vi "frontp_DO_replace_subpanel.vi"(8 "error in (no error)":errorcluster, 10 "changed_subpanel":refnum<vi>, 11 "front_panel in":refnum<class "front_panel.lvclass">) -> (0 "error out":errorcluster, 3 "front_panel out":refnum<class "front_panel.lvclass">)   [LabVIEW 2015, in "front_panel.lvclass"]
uses:
  front_panel.lvclass
  Hardware Class/hardware/hardware.lvclass
  hardware_caller_queue_numbers.ctl
  <vilib>/ActorFramework/Message Enqueuer/Message Enqueuer.lvclass/Message Enqueuer.ctl
  panel_class/panel.lvclass/panel.ctl
  stage_types.ctl
  Hardware Class/hardware_panel/Hardware_panel.lvclass
  Stage Class/Newport XPS/xps_panel/newport_xps_panel.lvclass
  Stage Class/Galvos_usb6212/galvo_panel/galvo_panel.lvclass
  Stage Class/Thorlabs Kinesis/thorlabs_panel/thorlabs_panel.lvclass
  Stage Class/MCL_3d200/mcl_panel.lvclass
  experiment_types.ctl
  Experiment/experiment_panel/Scan/scan_panel.lvclass
  Experiment/experiment_panel/2d_scan/scan_2d.lvclass
  Experiment/experiment_panel/PCFS/pcfs.lvclass
  detector_types.ctl
  Detector_Class/Picoquant/Hydraharp/hydraharp_panel/hydraharp_panel.lvclass
  Detector_Class/Picoquant/Picoharp/picoharp_panel/picoharp_panel.lvclass
  Detector_Class/Lightfield/lightfield_panel/lightfield_panel.lvclass
  <vilib>/ActorFramework/Message Enqueuer/Enqueue.vi
  <vilib>/ActorFramework/Message Priority Queue/Priority Enqueue.vi
  <vilib>/ActorFramework/Stop Msg/Stop Msg.lvclass
  panel_class/panel.lvclass
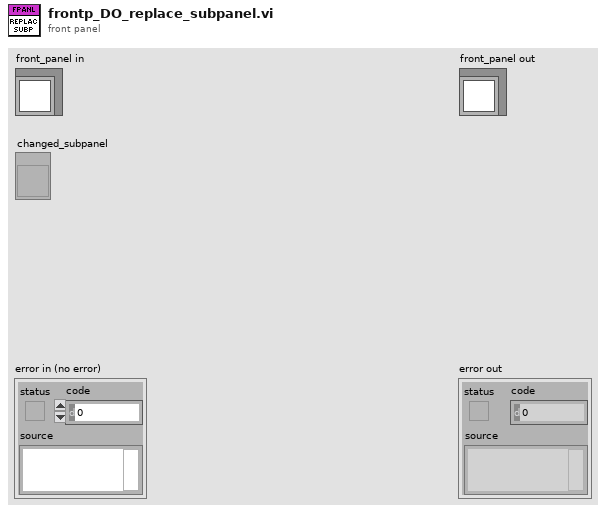
[diagram p1: front panel]
types:
  T1 = typedef "hardware_caller_queue_numbers.ctl" = enum16{"stage1", "stage2", "experiment", "detector"}
  T2 = typedef "stage_types.ctl" = enum16{"default", "Newport XPS", "Aerotech Ensemble", "Galvos", "Throlabs Kinesis", "MCL XYZ Piezo"}
  T3 = typedef "experiment_types.ctl" = enum16{"default", "PCFS", "Scan", "2D Galvo Scan"}
  T4 = typedef "detector_types.ctl" = enum16{"default", "Hydraharp", "Picoharp", "Lightfield"}
  T5 = typedef "ui_elements.ctl" = cluster{"map_xcursor":refnum<vi>, "map_ycursor":refnum<vi>}
  T6 = typedef "hardware_seqs.ctl" = refnum<queue>[]
  T7 = typedef "ui_plot_references.ctl" = cluster{"plots":refnum<vi>, "chart":refnum<vi>, "graph":refnum<vi>, "map":refnum<vi>, "XY Graph":refnum<vi>}
  T8 = typedef "ui_user_events.ctl" = cluster{"update_xy_graph":refnum<user-event>, "update_graph":refnum<user-event>, "update_chart":refnum<user-event>, "update_map":refnum<user-event>, "event_loop_stop":refnum<user-event>, "keep_map":refnum<user-event>}
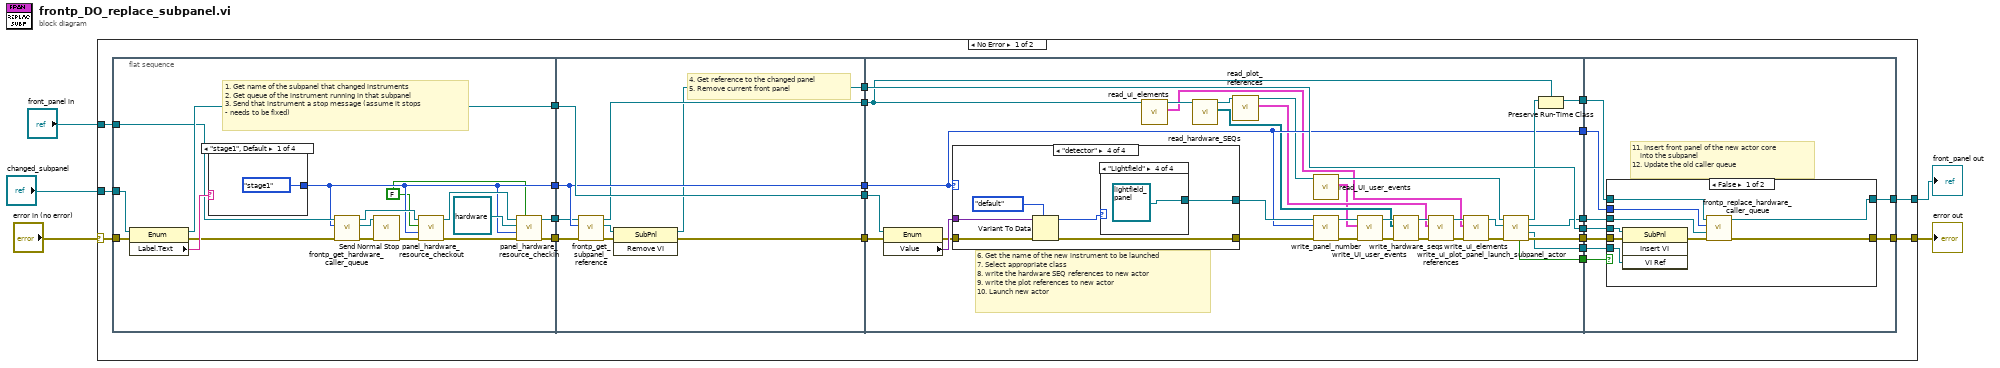
[diagram p0: block diagram]
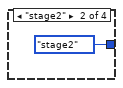
[diagram p2: hidden frame]
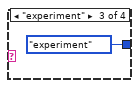
[diagram p3: hidden frame]
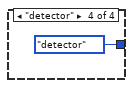
[diagram p4: hidden frame]
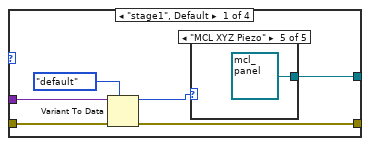
[diagram p5: hidden frame]
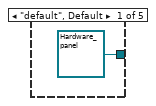
[diagram p6: hidden frame]
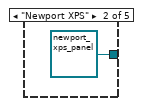
[diagram p7: hidden frame]
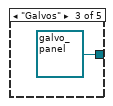
[diagram p8: hidden frame]
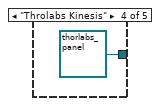
[diagram p9: hidden frame]
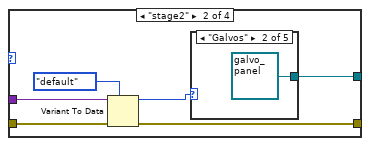
[diagram p10: hidden frame]
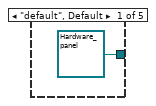
[diagram p11: hidden frame]
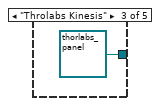
[diagram p12: hidden frame]
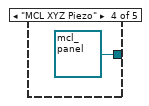
[diagram p13: hidden frame]
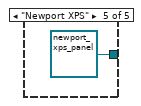
[diagram p14: hidden frame]
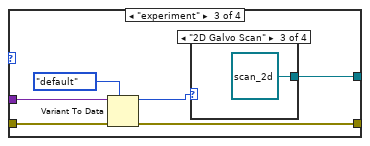
[diagram p15: hidden frame]
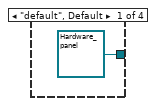
[diagram p16: hidden frame]
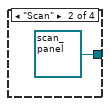
[diagram p17: hidden frame]
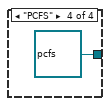
[diagram p18: hidden frame]
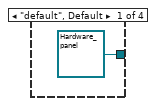
[diagram p19: hidden frame]
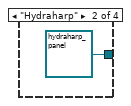
[diagram p20: hidden frame]
diagram:
  n1 = case shown="No Error" "error in (no error)" {
    selector: "error in (no error)" -> [w25 w153]
    tunnel: [w9 w153] -> w4
    tunnel: [w8 w152] -> w1
    tunnel: "front_panel in" -> [w24 w152]
    tunnel: "changed_subpanel" -> [w26 _]
    frame No Error {
      n2 = flat-sequence {
        tunnel: w26 -> [w43]
        tunnel: w25 -> [w42]
        tunnel: w24 -> [w37]
        tunnel: [w33] -> w23
        tunnel: [w30] -> w22
        tunnel: [w38] -> w21
        tunnel: [w28] -> w20
        tunnel: w23 -> [w55]
        tunnel: w22 -> [w53]
        tunnel: w21 -> [w56]
        tunnel: w20 -> [w54]
        tunnel: [w49] -> w19
        tunnel: [w52] -> w18
        tunnel: [w56] -> w17
        tunnel: [w54] -> w16
        tunnel: [w48] -> w15
        tunnel: w19 -> [w87]
        tunnel: w18 -> [w59]
        tunnel: w17 -> [w86]
        tunnel: w16 -> [w70]
        tunnel: w15 -> [w85]
        tunnel: [w82] -> w14
        tunnel: [w84] -> w13
        tunnel: [w85] -> w12
        tunnel: [w83] -> w11
        tunnel: [w70] -> w10
        tunnel: [w81] -> w7
        tunnel: [w79] -> w6
        tunnel: w14 -> [w140]
        tunnel: w13 -> [w139]
        tunnel: w12 -> [w138]
        tunnel: w11 -> [w137]
        tunnel: w10 -> [w136]
        tunnel: [w135] -> w9
        tunnel: [w134] -> w8
        tunnel: w7 -> [w133]
        tunnel: w6 -> [w132]
        frame #0 {
          w27 = FALSE ("Self?")
          # "1. Get name of the subpanel that changed instruments\n2. Get queue of the instrument running in that subpanel\n3. Send that instrument a stop message (assume it stops \n- needs to be fixed)"
          n3 = property class="Enum"(reference=w43, error in=w42) -> (reference out=w38:refnum<vi>, error out=w36:errorcluster, "Label.Text"=w41:string)
          n4 = case shown="\"stage1\", Default" w41 {
            tunnel: [hardware_caller_queue_numbers."stage1" ("hardware") hardware_caller_queue_numbers."stage2" ("hardware") hardware_caller_queue_numbers."experiment" ("hardware") hardware_caller_queue_numbers."detector" ("hardware")] -> w28
            frame "stage1", Default {
            }
            frame "stage2" {
            }
            frame "experiment" {
            }
            frame "detector" {
            }
          }
          n5 = call "frontp_get_hardware_caller_queue.vi"("error in (no error)"=w36, "hardware"=w28, "front_panel in"=w37) -> ("error out"=w40:errorcluster, "Nested Actor's Enqueuer"=w39:refnum<class "Message Enqueuer.lvclass">, "front_panel out"=w32:refnum<class "front_panel.lvclass">)  [unwired: 6 in]
          n6 = call <vilib>:"Send Normal Stop.vi"("error in (no error)"=w40, "Message Enqueuer"=w39) -> ("error out"=w35:errorcluster)  [unwired: 9 in]
          n7 = call "panel_hardware_resource_checkout.vi"("error in (no error)"=w35, "panel_number"=w28, "Self?"=w27, "panel in"=w32) -> ("error out"=w34:errorcluster, "panel out"=w31:refnum<class "front_panel.lvclass">)  [unwired: 4 in, 2 out]
          n8 = call "panel_hardware_resource_checkin.vi"("Self"=w27, "error in (no error)"=w34, "panel_number"=w28, "hardware.lvclass"=refnum<class "hardware.lvclass"> refnum, "panel in"=w31) -> ("error out"=w33:errorcluster, "panel out"=w30:refnum<class "front_panel.lvclass">)  [unwired: 5 in]
        }
        frame #1 {
          # "4. Get reference to the changed panel\n5. Remove current front panel"
          n9 = call "frontp_get_subpanel_reference.vi"("error in (no error)"=w55, "hardware"=w54, "front_panel in"=w53) -> ("error out"=w50:errorcluster, "subpanel"=w51:refnum<vi>, "front_panel out"=w52:refnum<class "front_panel.lvclass">)  [unwired: 6 in]
          n10 = invoke class="SubPnl" method="Remove VI"(reference=w51, error in=w50) -> (reference out=w48:refnum<vi>, error out=w49:errorcluster)  [unwired: 1 in, 1 out]
        }
        frame #2 {
          # "6. Get the name of the new instrument to be launched\n7. Select appropriate class\n8. write the hardware SEQ references to new actor\n9. write the plot references to new actor\n10. Launch new actor"
          n11 = property class="Enum"(reference=w86, error in=w87) -> (error out=w88:errorcluster, "Value"=w89:variant)  [unwired: 1 out]
          n12 = case shown="\"detector\"" w70 {
            tunnel: w89 -> [w95 w104 w117 w127]
            tunnel: [w92 w102 w113 w122] -> w72
            tunnel: w88 -> [w91 w103 w115 w126]
            tunnel: [w90 w101 w112 w125] -> w74
            frame "stage1", Default {
              n13 = Variant To Data(error in=w91, type=stage_types."default" ("stage1"), Variant=w95) -> (data=w93:T2, error out=w90:errorcluster)
              n14 = case shown="\"MCL XYZ Piezo\"" w93 {
                tunnel: [refnum<class "Hardware_panel.lvclass"> refnum ("Hardware_panel.lvclass") refnum<class "newport_xps_panel.lvclass"> refnum ("newport_xps_panel.lvclass") refnum<class "galvo_panel.lvclass"> refnum ("galvo_panel.lvclass") refnum<class "thorlabs_panel.lvclass"> refnum ("thorlabs_panel.lvclass") refnum<class "mcl_panel.lvclass"> refnum ("mcl_panel.lvclass")] -> w92
                frame "default", Default {
                }
                frame "Newport XPS" {
                }
                frame "Galvos" {
                }
                frame "Throlabs Kinesis" {
                }
                frame "MCL XYZ Piezo" {
                }
              }
            }
            frame "stage2" {
              n15 = Variant To Data(error in=w103, type=stage_types."default" ("stage1"), Variant=w104) -> (data=w105:T2, error out=w101:errorcluster)
              n16 = case shown="\"Galvos\"" w105 {
                tunnel: [refnum<class "Hardware_panel.lvclass"> refnum ("Hardware_panel.lvclass") refnum<class "galvo_panel.lvclass"> refnum ("galvo_panel.lvclass") refnum<class "thorlabs_panel.lvclass"> refnum ("thorlabs_panel.lvclass") refnum<class "mcl_panel.lvclass"> refnum ("mcl_panel.lvclass") refnum<class "newport_xps_panel.lvclass"> refnum ("newport_xps_panel.lvclass")] -> w102
                frame "default", Default {
                }
                frame "Galvos" {
                }
                frame "Throlabs Kinesis" {
                }
                frame "MCL XYZ Piezo" {
                }
                frame "Newport XPS" {
                }
              }
            }
            frame "experiment" {
              n17 = Variant To Data(error in=w115, type=experiment_types."default" ("experiment"), Variant=w117) -> (data=w114:T3, error out=w112:errorcluster)
              n18 = case shown="\"2D Galvo Scan\"" w114 {
                tunnel: [refnum<class "Hardware_panel.lvclass"> refnum ("Hardware.lvclass") refnum<class "scan_panel.lvclass"> refnum ("scan_panel.lvclass") refnum<class "scan_2d.lvclass"> refnum ("scan_2d.lvclass") refnum<class "pcfs.lvclass"> refnum ("pcfs.lvclass")] -> w113
                frame "default", Default {
                }
                frame "Scan" {
                }
                frame "2D Galvo Scan" {
                }
                frame "PCFS" {
                }
              }
            }
            frame "detector" {
              n19 = Variant To Data(error in=w126, type=detector_types."default" ("detector"), Variant=w127) -> (data=w123:T4, error out=w125:errorcluster)
              n20 = case shown="\"Lightfield\"" w123 {
                tunnel: [refnum<class "Hardware_panel.lvclass"> refnum ("Hardware.lvclass") refnum<class "hydraharp_panel.lvclass"> refnum ("hydraharp.lvclass") refnum<class "picoharp_panel.lvclass"> refnum ("picoharp_panel.lvclass") refnum<class "lightfield_panel.lvclass"> refnum ("lightfield_panel.lvclass")] -> w122
                frame "default", Default {
                }
                frame "Hydraharp" {
                }
                frame "Picoharp" {
                }
                frame "Lightfield" {
                }
              }
            }
          }
          n21 = call "read_ui_elements.vi"("panel in"=w59) -> ("ui_elements"=w57:T5, "panel out"=w58:refnum<class "front_panel.lvclass">)  [unwired: 8 in, 1 out]
          n22 = call "read_hardware_SEQs.vi"("panel in"=w58) -> ("hardware_SEQs"=w67:T6, "panel out"=w69:refnum<class "front_panel.lvclass">)  [unwired: 8 in, 1 out]
          n23 = call "read_plot_references.vi"("panel in"=w69) -> ("plot_references"=w66:T7, "panel out"=w68:refnum<class "front_panel.lvclass">)  [unwired: 8 in, 1 out]
          n24 = call "read_UI_user_events.vi"("panel in"=w68) -> ("ui_user_events"=w65:T8, "panel out"=w64:refnum<class "front_panel.lvclass">)  [unwired: 8 in, 1 out]
          n25 = call "write_panel_number.vi"("error in (no error)"=w74, "panel_number"=w70, "panel in"=w72) -> ("error out"=w73:errorcluster, "panel out"=w71:refnum<class "panel.lvclass">)  [unwired: 7 in]
          n26 = call "write_UI_user_events.vi"("error in (no error)"=w73, "ui_events"=w65, "panel in"=w71) -> ("error out"=w76:errorcluster, "panel out"=w75:refnum<class "panel.lvclass">)  [unwired: 7 in]
          n27 = call "write_hardware_seqs.vi"("error in (no error)"=w76, "hardware_SEQs"=w67, "panel in"=w75) -> ("error out"=w77:errorcluster, "panel out"=w78:refnum<class "panel.lvclass">)  [unwired: 7 in]
          n28 = call "write_ui_plot_references.vi"("error in (no error)"=w77, "plot_references"=w66, "panel in"=w78) -> ("error out"=w63:errorcluster, "panel out"=w61:refnum<class "panel.lvclass">)  [unwired: 7 in]
          n29 = call "write_ui_elements.vi"("error in (no error)"=w63, "ui_elements"=w57, "panel in"=w61) -> ("error out"=w62:errorcluster, "panel out"=w60:refnum<class "panel.lvclass">)  [unwired: 7 in]
          n30 = call-dynamic "panel_launch_subpanel_actor.vi"("error in (no error)"=w62, "nested_panel"=w60, "caller_panel"=w64) -> ("error out"=w84:errorcluster, "subpanel_reference"=w82:refnum<vi>, "Nested Actor's Enqueuer"=w83:refnum<class "Message Enqueuer.lvclass">, "Caller Actor out"=w80:refnum<class "panel.lvclass">, "timed out?"=w81:bool)  [unwired: 4 in]
          n31 = Preserve Run-Time Class(object in=w80, 2:w59) -> (object out=w79:refnum<class "front_panel.lvclass">)  [unwired: 1 in, 1 out]
        }
        frame #3 {
          # "11. Insert front panel of the new actor core\n    into the subpanel\n12. Update the old caller queue"
          n32 = case shown="False" w133 {
            tunnel: w137 -> [w144 _]
            tunnel: w140 -> [w148 _]
            tunnel: w138 -> [w149 _]
            tunnel: w139 -> [w147 w151]
            tunnel: w136 -> [w145 _]
            tunnel: [w143 w151] -> w135
            tunnel: [w142 w150] -> w134
            tunnel: w132 -> [w141 w150]
            frame False {
              n33 = invoke class="SubPnl" method="Insert VI"(reference=w149, error in=w147, "VI Ref"=w148) -> (error out=w146:errorcluster)  [unwired: 1 in, 3 out]
              n34 = call "frontp_replace_hardware_caller_queue.vi"("error in (no error)"=w146, "Nested Actor's Enqueuer"=w144, "hardware"=w145, "front_panel in"=w141) -> ("error out"=w143:errorcluster, "front_panel out"=w142:refnum<class "front_panel.lvclass">)  [unwired: 6 in]
            }
            frame True {
            }
          }
        }
      }
    }
    frame Error {
    }
  }
  "error out" <- w4
  "front_panel out" <- w1
